vi "SOUR_POW_CORR_COLL_ITER_COUN.vi"(0 "VISA IN":refnum<visa-resource-name>, 5 "error in":errorcluster, 7 "Max number of readings":i32) -> (14 "VISA Out":refnum<visa-resource-name>, 19 "error out":errorcluster)   [LabVIEW 2018, in "PNA-X.lvlib"]
doc: "SOURce:POWer:CORRection:COLLect:ITERation[:COUNt] <num> \n(Read-Write) This command, along with SOUR:POW:CORR:COLL:ITER:NTOL describes the \nnumber of ADUSTMENTS to make to the source power. \nSets the maximum number of readings to take at each data point for iterating the source power. Power \nREADINGS (performed by SOUR:POW:CORR:COLL:AVER:COUNT and \nSOUR:POW:CORR:COLL:AVER:NTOLerance) will continue to be made, and source power \nadjusted, until the measurement is within the iteration tolerance value or this max number of \nmeasurements has been met. The last value is the valid measurement for that data point. \nLearn more. \nParameters \n<num> Maximum number of readings. Choose any number between 1 and 100. \nExamples SOUR:POW:CORR:COLL:ITER 2 \nsource:power:correction:collect:iteration 3 \nQuery Syntax SOURce:POWer:CORRection:COLLect:ITERation[:COUNt]? \nReturn Type Numeric \nDefault 1"
uses:
  PNA-X.lvlib
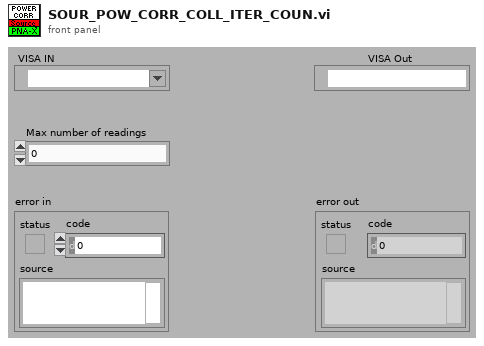
[diagram p1: front panel]
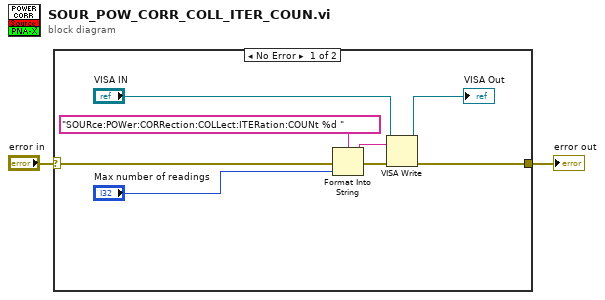
[diagram p0: block diagram]
diagram:
  n1 = case shown="No Error" "error in" {
    selector: "error in" -> [w10 w11]
    tunnel: [w5 w11] -> w1
    frame No Error {
      n2 = Format Into String(format string="SOURce:POWer:CORRection:COLLect:ITERation:COUNt %d " ("Cmdline"), error in=w10, "Max number of readings") -> (resulting string=w8:string, error out=w9:errorcluster)  [unwired: 1 in]
      n3 = VISA Write(VISA resource name="VISA IN", write buffer=w8, error in (no error)=w9) -> (VISA resource name out=→"VISA Out":refnum<visa-resource-name>, error out=w5:errorcluster)  [unwired: 1 out]
    }
    frame Error {
    }
  }
  "error out" <- w1
